vi "Format_Actions_String.vi"(9 "z action":string, 10 "y action":string, 11 "x action":string) -> (3 "String":string)   [LabVIEW 2013, in "Mercury iXX.lvlib"]
uses:
  <instrlib>/Mercury iXX/Mercury iXX.lvlib
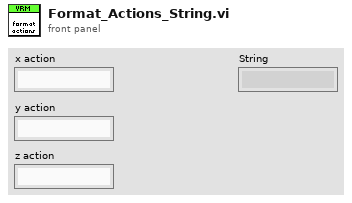
[diagram p1: front panel]
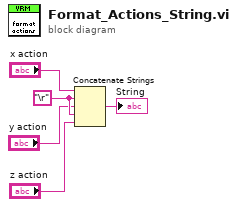
[diagram p0: block diagram]
diagram:
  w4 = "\r"
  n1 = Concatenate Strings("x action", w4, "y action", w4, "z action") -> (→"String":string)
